vi "StartCW.vi"(0 "FPGA Reference":refnum<k20>, 1 "Enum":T1, 2 "Enable PA":enum8{"0", "1"}(ring), 5 "CW Freq (Hz)":u32=1, 7 "Freq Offset (Hz)":i32=1, 9 "Pwr Reduction (dB/2)":i8=1, 11 "Error In":errorcluster, 12 "Resp Timeout (ms)":i32 min=0, 13 "CW Type":enum8{"0", "1", "2"}(ring)) -> (6 "Start CW OK":bool, 8 "Received Text":string, 15 "Error Out":errorcluster)   [LabVIEW 2018]
uses:
  Resources_Test/UART/ControlTestSlot.ctl
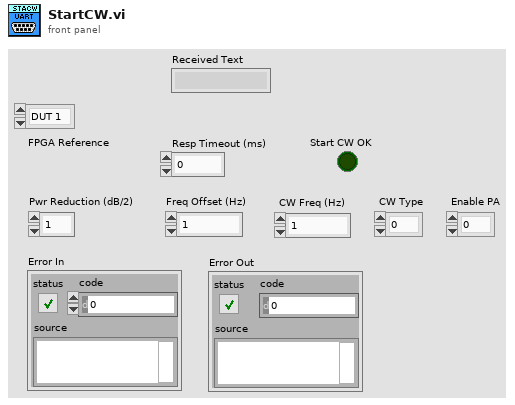
[diagram p1: front panel]
types:
  T1 = typedef "ControlTestSlot.ctl" = enum16{"DUT 1", "DUT 2"}
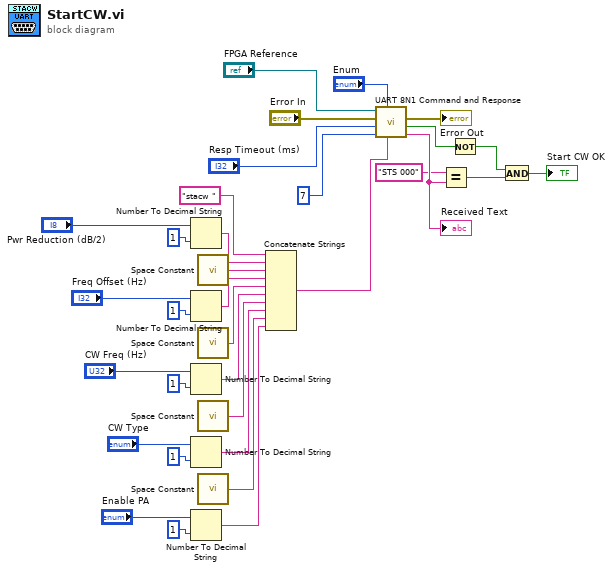
[diagram p0: block diagram]
diagram:
  n1 = Number To Decimal String(number="Pwr Reduction (dB/2)", width (-)=i16 1) -> (decimal integer string=w27:string)
  n2 = Number To Decimal String(number="Freq Offset (Hz)", width (-)=i16 1) -> (decimal integer string=w23:string)
  n3 = Number To Decimal String(number="CW Freq (Hz)", width (-)=i16 1) -> (decimal integer string=w19:string)
  n4 = Number To Decimal String(number="CW Type", width (-)=i16 1) -> (decimal integer string=w15:string)
  n5 = Number To Decimal String(number="Enable PA", width (-)=i16 1) -> (decimal integer string=w11:string)
  n6 = call <vilib>:"Space Constant.vi"() -> ("String"=w26:string)
  n7 = call <vilib>:"Space Constant.vi"() -> ("String"=w22:string)
  n8 = call <vilib>:"Space Constant.vi"() -> ("String"=w18:string)
  n9 = call <vilib>:"Space Constant.vi"() -> ("String"=w12:string)
  n10 = Concatenate Strings("stacw " ("Text to Send"), w27, w26, w23, w22, w19, w18, w15, w12, w11) -> (w5:string)
  n11 = call "UART 8N1 Command and Response.vi"("Text to Send"=w5, "Active Dut"="Enum", "Response Size (char)"=u32 7, "Response Timeout (ms)"="Resp Timeout (ms)", "Error In"="Error In", "FPGA VI Reference In"="FPGA Reference") -> ("Received Text"=w2:string, "Timeout Flag"=w3:bool, "Error Out"=→"Error Out":errorcluster)  [unwired: 1 in, 2 out]
  "Received Text" <- w2
  n12 = Equal?(x="STS 000" ("y"), y=w2) -> (x = y?=w31:bool)
  n13 = Not(x=w3) -> (.not. x?=w33:bool)
  n14 = And(x=w33, y=w31) -> (x .and. y?=→"Start CW OK":bool)
